vi "Acquire_Prototype2.vi"() -> ()   [LabVIEW 2013, in "MagSpec_Bella.lvclass"]
uses:
  MagSpec_Bella.lvclass
  MagSpec_Bella.lvclass/MagSpec_Bella.ctl
  <vilib>/vision/NI_Vision_Development_Module.lvlib
  MagSpecCamera.lvclass
panel:
  out "get Images":u32
  out "time":u32[](array[numeric])
  out "total time":u32
  in  "Sim Image Index 2":i32=3
  in  "B [T] in":dbl=0.63
  out "Numeric 3":i32
  in  "stop":bool
  out "Image Out":T1(plugin-control)
  out "Empty Image":bool[](array[boolean])
  out "error out":errorcluster
  out "Sum Y":cluster{"Momentum [MeV/C]":dbl[], dbl[]}[](graph)
  in  "MagSpec_Bella.lvclass":refnum<class "MagSpec_Bella.lvclass">
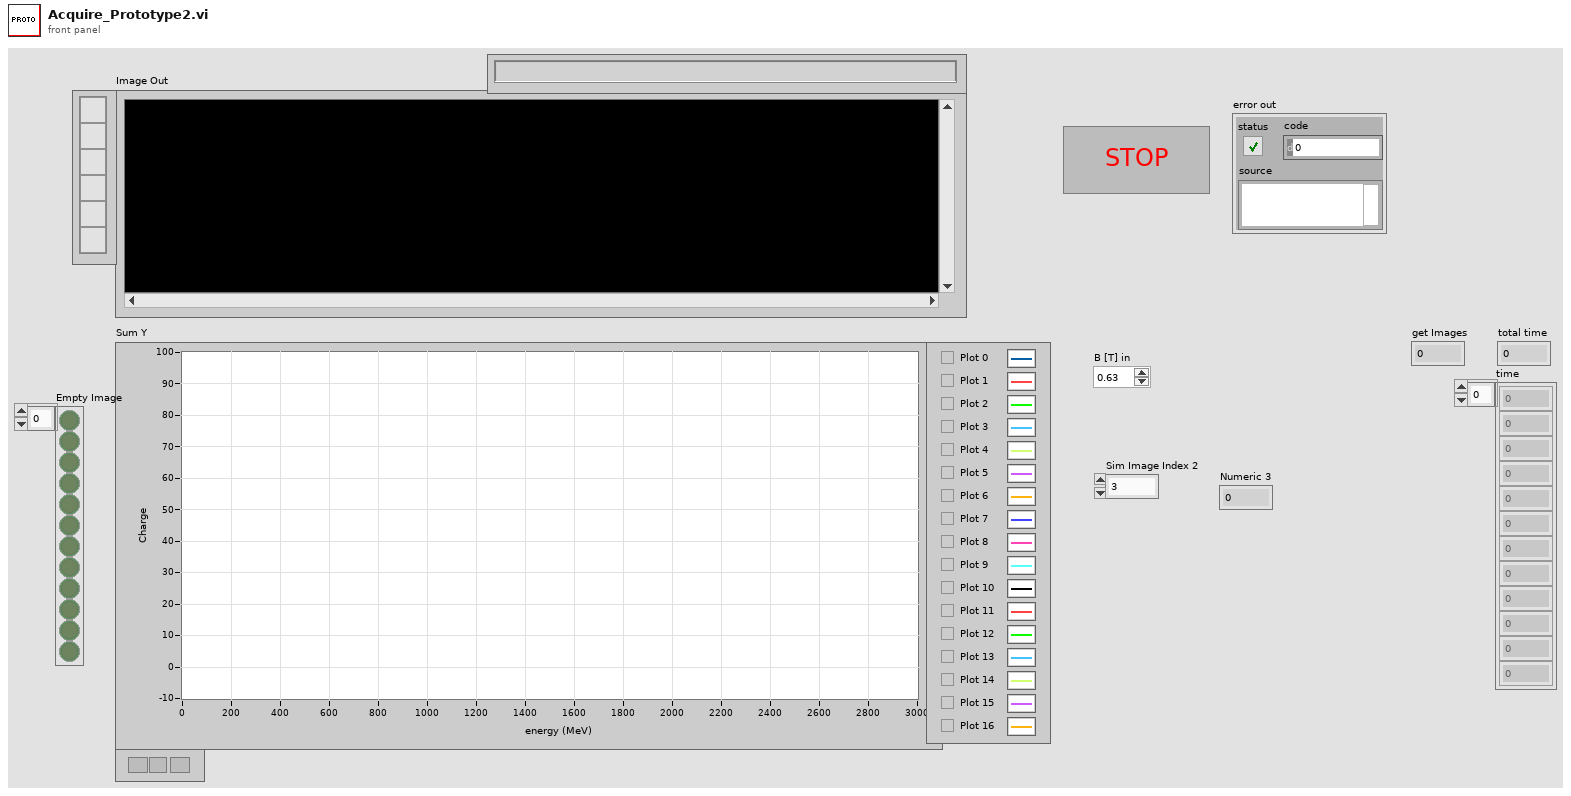
[diagram p1: front panel]
types:
  T1 = typedef "IMAQ Image.ctl" = refnum<image>
  T2 = typedef "Image Type" = u32
  T3 = typedef "CameraSettings_File.ctl" = cluster{"FOV [mm]":dbl, "Left edge [mm]":dbl, "ROI Y offset":dbl, "ROI height":dbl, "ROI X offset":dbl, "ROI width":dbl, "Y center pixel":dbl, "Y Start":dbl, "Y End":dbl, "X Start":dbl, "X End":dbl, "rot [deg]":dbl}
  T4 = typedef "OneTimeCalculation.ctl" = cluster{"first Pixel pos [m]":dbl, "Pixel Size [mm]":dbl, "forward":T5}
  T5 = typedef "OnOffTypeDef.ctl" = enum16{"off", "on"}
  T6 = typedef "2D.ctl" = cluster{"dp":dbl[][], "chargeCompensation":dbl[][], "angle":dbl[][], "Momentum":dbl[][]}
  T7 = typedef "finalCalib--Cluster.ctl" = cluster{"X":dbl[][], "xi":dbl[][], "delta momentum":dbl, "Y":dbl[][], "yi":dbl[][], "angle (Y)":dbl[], "delta angle":dbl, "scale delta angle":dbl, "intraX":dbl, "intraY":dbl, "mask":dbl[][]}
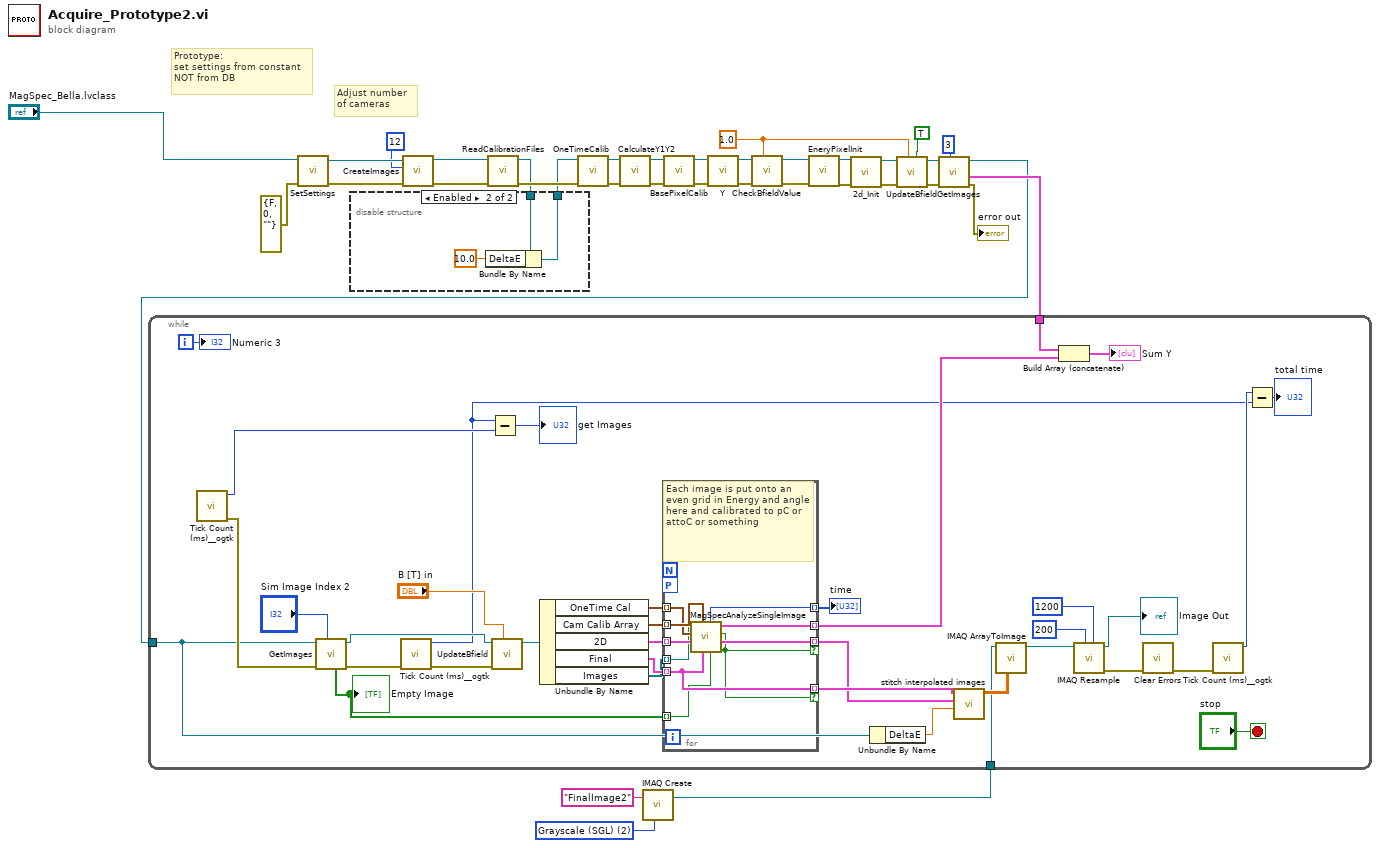
[diagram p0: block diagram]
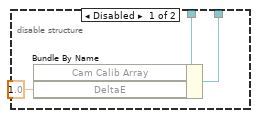
[diagram p2: hidden frame]
diagram:
  w3 = 1.0 ("B [T] in")
  w6 = T2 2 items=["Grayscale (U8)", "Grayscale (I16)", "Grayscale (SGL)", "Complex (CSG)", "RGB (U32)", "HSL (U32)", "RGB (U64)", "Grayscale (U16)"] ("Image Type")
  # "Adjust number\nof cameras"
  # "Prototype:\nset settings from constant\nNOT from DB"
  n1 = call "SetSettings.vi"("error in (no error)"=errorcluster {"status"=FALSE, "code"=0, "source"=""} ("error out"), "MagSpec_Bella in"="MagSpec_Bella.lvclass") -> ("error out"=w30:errorcluster, "MagSpec_Bella out"=w32:refnum<class "MagSpec_Bella.lvclass">)  [unwired: 8 in]
  n2 = call "CreateImages.vi"("error in (no error)"=w30, "Numeric"=12, "MagSpec_Bella in"=w32) -> ("error out"=w29:errorcluster, "MagSpec_Bella out"=w14:refnum<class "MagSpec_Bella.lvclass">)  [unwired: 7 in]
  n3 = call "ReadCalibrationFiles.vi"("error in (no error)"=w29, "MagSpec_Bella in"=w14) -> ("error out"=w28:errorcluster, "MagSpec_Bella out"=w13:refnum<class "MagSpec_Bella.lvclass">)  [unwired: 8 in]
  n4 = disable-structure shown="Enabled" {
    disable-tunnel: w13 -> [w37 w41]
    disable-tunnel: [w36 w40] -> w12
    frame Disabled {
      n5 = Bundle By Name(cluster=w37, "DeltaE"=1.0) -> (w36:refnum<class "MagSpec_Bella.lvclass">, "Cam Calib Array"=w38:T3[])
    }
    frame Enabled {
      n6 = Bundle By Name(cluster=w41, "DeltaE"=10.0) -> (w40:refnum<class "MagSpec_Bella.lvclass">)
    }
  }
  n7 = call "OneTimeCalib.vi"("error in"=w28, "MagSpec_Bella in"=w12) -> ("error out"=w23:errorcluster, "MagSpec_Bella out"=w24:refnum<class "MagSpec_Bella.lvclass">)  [unwired: 8 in]
  n8 = call "CalculateY1Y2.vi"("error in"=w23, "MagSpec_Bella in"=w24) -> ("error out"=w21:errorcluster, "MagSpec_Bella out"=w22:refnum<class "MagSpec_Bella.lvclass">)  [unwired: 8 in]
  n9 = call "IMAQ Create"("Image Name"="FinalImage2", "Image Type"=w6) -> ("New Image"=w1:T1)  [unwired: 3 in, 1 out]
  n10 = call "BasePixelCalib.vi"("error in (no error)"=w21, "MagSpec_Bella in"=w22) -> ("error out"=w18:errorcluster, "MagSpec_Bella out"=w20:refnum<class "MagSpec_Bella.lvclass">)  [unwired: 8 in]
  n11 = call "Y.vi"("error in (no error)"=w18, "MagSpec_Bella in"=w20) -> ("error out"=w17:errorcluster, "MagSpec_Bella out"=w19:refnum<class "MagSpec_Bella.lvclass">)  [unwired: 8 in]
  n12 = call "CheckBfieldValue .vi"("B [T] new"=w3, "MagSpec_Bella in"=w19) -> ("MagSpec_Bella out"=w7:refnum<class "MagSpec_Bella.lvclass">)  [unwired: 8 in, 1 out]
  n13 = call "EneryPixelInit.vi"("error in (no error)"=w17, "MagSpec_Bella in"=w7) -> ("error out"=w8:errorcluster, "MagSpec_Bella out"=w9:refnum<class "MagSpec_Bella.lvclass">)  [unwired: 8 in]
  n14 = call "2d_Init.vi"("error in (no error)"=w8, "MagSpec_Bella in"=w9) -> ("error out"=w25:errorcluster, "MagSpec_Bella out"=w26:refnum<class "MagSpec_Bella.lvclass">)  [unwired: 8 in]
  n15 = call "UpdateBfield.vi"("Force upodate (F)"=TRUE ("Force upodate"), "B [T] in"=w3, "error in (no error)"=w25, "MagSpec_Bella in"=w26) -> ("error out"=w27:errorcluster, "MagSpec_Bella out"=w34:refnum<class "MagSpec_Bella.lvclass">)  [unwired: 6 in]
  n16 = call "GetImages.vi"("Sim Image Index"=3, "error in (no error)"=w27, "MagSpec_Bella in"=w34) -> ("error out"=→"error out":errorcluster, "output cluster"=w11:cluster{dbl[], dbl[]}[], "MagSpec_Bella out"=w2:refnum<class "MagSpec_Bella.lvclass">)  [unwired: 5 in, 1 out]
  n17 = while {
    tunnel: w11 -> [w72]
    tunnel: w2 -> [w44]
    tunnel: w1 -> [w42]
    i -> [w66]
    stop <- "stop" stop-if-true
    n18 = call <userlib>:"Tick Count (ms)__ogtk.vi"() -> ("error out"=w48:errorcluster, "millisecond timer value"=w47:u32)  [unwired: 10 in]
    n19 = call "GetImages.vi"("Sim Image Index"="Sim Image Index 2", "error in (no error)"=w48, "MagSpec_Bella in"=w44) -> ("error out"=w50:errorcluster, "MagSpec_Bella out"=w64:refnum<class "MagSpec_Bella.lvclass">, "Empty Image"=w60:bool[])  [unwired: 5 in, 1 out]
    "Empty Image" <- w60
    n20 = call <userlib>:"Tick Count (ms)__ogtk.vi"("error in (no error)"=w50) -> ("error out"=w49:errorcluster, "millisecond timer value"=w45:u32)  [unwired: 9 in]
    n21 = Subtract(x=w45, y=w47) -> (x-y=→"get Images":u32)
    n22 = call "UpdateBfield.vi"("B [T] in"="B [T] in", "error in (no error)"=w49, "MagSpec_Bella in"=w64) -> ("MagSpec_Bella out"=w68:refnum<class "MagSpec_Bella.lvclass">)  [unwired: 7 in, 1 out]
    n23 = Unbundle By Name(w68) -> ("OneTime Cal"=w73:T4[], "Cam Calib Array"=w74:T3[], "2D"=w77:T6[], "Final"=w76:T7[], "Images"=w75:T1[])
    n24 = for {
      tunnel: w77 -> [w87] mode=indexing
      tunnel: w76 -> [w82] mode=indexing
      tunnel: w75 -> [w83] mode=indexing
      tunnel: w74 -> [w86] mode=indexing
      tunnel: w73 -> [w85] mode=indexing
      tunnel: [w84] -> w71 mode=indexing
      tunnel: [w82] -> w70 mode=indexing if=w80
      tunnel: [w81] -> w69 mode=indexing if=w80
      workers-P: _ -> [_]
      tunnel: w60 -> [w79] mode=indexing
      tunnel: [w78] -> w51 mode=indexing
      # "Each image is put onto an even grid in Energy and angle here and calibrated to pC or attoC or something"
      n25 = call "MagSpecAnalyzeSingleImage.vi"("empty image"=w79, "Cluster in"=w82, "Camera Settings"=w86, "2D"=w87, "One time calculation"=w85, "Refnum in"=w83) -> ("Cluster out"=w81:cluster{dbl[][]}, "Boolean"=w80:bool, "spec cluster 2"=w84:cluster{"Momentum [MeV/C]":dbl[], dbl[]}, "time: 2Dinter"=w78:u32)  [unwired: 2 in]
    }
    "time" <- w51
    n26 = Unbundle By Name(w44) -> ("DeltaE"=w43:dbl)
    n27 = call "stitch interpolated images.vi"("DeltaE"=w43, "Array of images to stitch"=w69, "calib \"final\""=w70) -> ("stitched array image"=w57:sgl[][])  [unwired: 8 in]
    n28 = call "IMAQ ArrayToImage"("Image Pixels (Float)"=w57, "Image"=w42) -> ("Image Out"=w56:T1)  [unwired: 8 in, 1 out]
    n29 = Build Array (concatenate)(w72, w71) -> (→"Sum Y":cluster{"Momentum [MeV/C]":dbl[], dbl[]}[])
    n30 = call "IMAQ Resample"("X Resolution"=1200, "Y Resolution"=200, "Image Src"=w56) -> ("error out"=w53:errorcluster, "Image Dst Out"=→"Image Out":T1)  [unwired: 7 in]
    n31 = call <vilib>:"Clear Errors.vi"("error in (no error)"=w53) -> ("error out"=w62:errorcluster)  [unwired: 6 in]
    n32 = call <userlib>:"Tick Count (ms)__ogtk.vi"("error in (no error)"=w62) -> ("millisecond timer value"=w59:u32)  [unwired: 9 in, 1 out]
    n33 = Subtract(x=w59, y=w45) -> (x-y=→"total time":u32)
    "Numeric 3" <- w66
  }
